vi "AlliGator Phasor Ratio Step.vi"(4 "Interactive?":bool, 6 "Time Stamp":dbl, 7 "Current Phasor Refnum":refnum<vi>, 8 "Error In":errorcluster, 10 "Phasor Ratio Parameters":T2, 11 "Registered Events Ctrl Refnums":T1) -> (0 "Error Out":errorcluster, 3 "Notebook String":string)   [LabVIEW 2021, in "AlliGator Phasor Ratio.lvlib"]
doc: "Computes phasor ratio and updates graphs."
uses:
  AlliGator Phasor Ratio.lvlib
  AlliGator Phasor Ratio Parameters.ctl
  Phasor/Phasor (g, s).ctl
  GUI/AlliGator Registered Events Ctrl Refnums.ctl
  Settings/AlliGator Settings List.ctl
  Graphs/XY Graph/XY Graph Plot Shift Parameters.ctl
  Graphs/XY Graph/XY Graph Plot Shift Method.ctl
  Phasor/Phasor Ratio Type.ctl
  Phasor/Phasor Standard Deviation Options.ctl
  Phasor/Phasor.lvlib
  Graphs/XY Graph/XY Graph Add-Ons.lvlib
  Settings/AlliGator Settings.lvlib
  Decay Analysis/Decay Preprocessing/AlliGator Decay Preprocessing.lvlib
  GUI/AlliGator GUI.lvlib
panel:
  in  "Data":variant
  # "see the AlliGator License on the block diagram (Ctrl+E or Window:Show Block Diagram)"
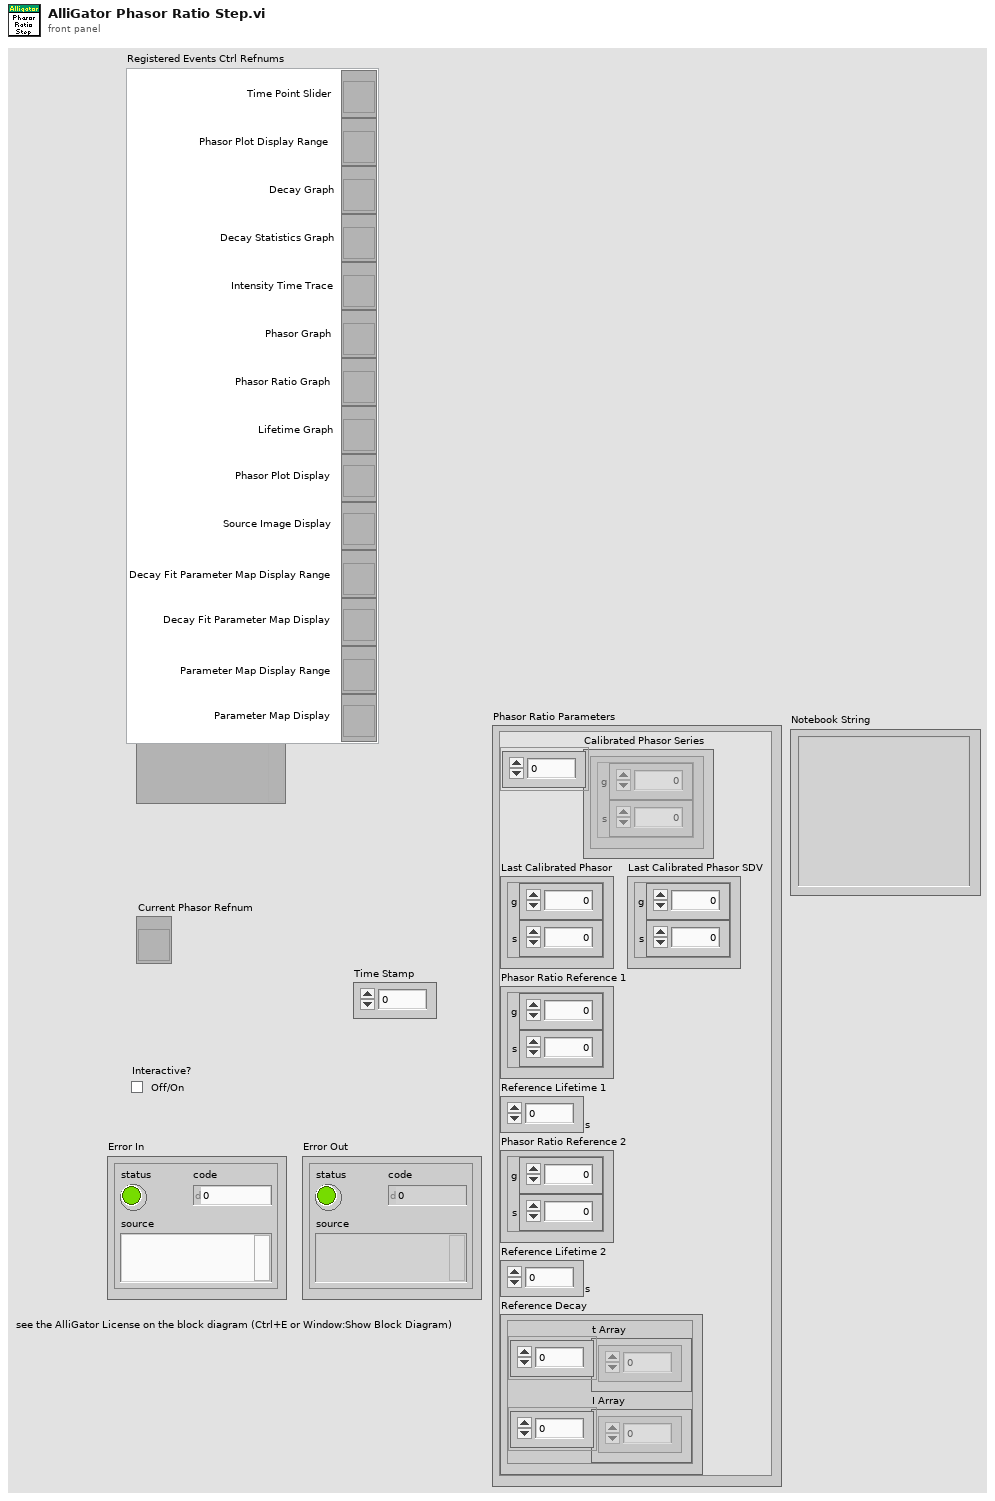
[diagram p1: front panel]
types:
  T1 = typedef "AlliGator GUI.lvlib/AlliGator Registered Events Ctrl Refnums.ctl" = cluster{"Time Point Slider":refnum<vi>, "Phasor Plot Display Range":refnum<vi>, "Decay Graph":refnum<vi>, "Decay Statistics Graph":refnum<vi>, "Intensity Time Trace":refnum<vi>, "Phasor Graph":refnum<vi>, "Phasor Ratio Graph":refnum<vi>, "Lifetime Graph":refnum<vi>, "Phasor Plot Display":refnum<vi>, "Source Image Display":refnum<vi>, "Decay Fit Parameter Map Display Range":refnum<vi>, "Decay Fit Parameter Map Display":refnum<vi>, "Parameter Map Display Range":refnum<vi>, "Parameter Map Display":refnum<vi>}
  T2 = typedef "AlliGator Phasor Ratio.lvlib/AlliGator Phasor Ratio Parameters.ctl" = cluster{"Calibrated Phasor Series":T3[], "Last Calibrated Phasor":T3, "Phasor Ratio Reference 1":T3, "Reference Lifetime 1":dbl[unit], "Phasor Ratio Reference 2":T3, "Reference Lifetime 2":dbl[unit], "Reference Decay":cluster{"t Array":dbl[], "I Array":dbl[]}, "Last Calibrated Phasor SDV":T3}
  T3 = typedef "Phasor.lvlib/Phasor (g, s).ctl" = cluster{"g":dbl, "s":dbl}
  T4 = typedef "XY Graph Add-Ons.lvlib/XY Graph Plot Shift Parameters.ctl" = cluster{"Type":T5, "Shift":dbl[unit], "Threshold":dbl, "Rotate":bool}
  T5 = typedef "XY Graph Add-Ons.lvlib/XY Graph Plot Shift Method.ctl" = enum16{"Default", "CFD", "Threshold", "Cross-Correlation"}
  T6 = typedef "AlliGator Settings.lvlib/AlliGator Settings List.ctl" = enum16{"GUI:Visible Settings Tab", "GUI:Last Run Version", "Source Image:Use Image Histogram for Contrast", "Source Image:Low Count Pixels Rejection Options", "Source Image:High Count Pixels Rejection Options", "Source Image:Use Image Brightness", "Source Image:Blend Overlay with Image Background", "Source Image:Use Fixed ROI Diameter", "Source Image:ROI Diameter", "Source Image:ROI Center Color", "Source Image:Peak Threshold", "Source Image:Intensity Threshold", "Source Image:Image Binning Options", "Source Image:Image Smoothing Options", "Source Image:Image Histogram Active", "Source Image:Invert Binary Mask", "Source Image:Hot Pixel Removal", "Source Image:Overlay Analyzed ROI Center", "Source Image:Auto-Adjust Contrast", "Source Image:Histogram Lower Percentile", "Source Image:Histogram Upper Percentile", "Source Image:Save Source Image", "Source Image:Scale Bar Options", "Source Image:Image Resolution (Pixel Size)", "Source Image:Flatfield Correction", "Source Image:Show Dead Left Columns Correction", "Source Image:Dead Left Columns Correction", "Source Image:Image Pre-Processing Operations Order", "Source Image:Overlay ROI Median", "Source Image:Median Overlay Color", "Data Information:Gate Width", "Data Information:Nanotime Gate Separation", "Data Information:Macrotime Gate Separation", "Data Information:Gate Step", "Data Information:# Gates", "Data Information:Gate Image Exposure", "Data Information:Gate Image Integration", "Data Information:Gates to Skip", "Data Information:Gates to Keep", "Data Information:Define Gates to", "Data Information:Channel Name", "Data Information:Available Channel Names", "Data Information:Channel Arithmetic", "Data Information:Background File Subtraction", "Data Information:Background File", "Data Information:Background Scaling Factor", "Data Information:Background Pile-up Correction", "Data Information:Background Pixel Well Capacity", "Data Information:Laser Period", "Data Information:SYNC Period", "Data Information:Pile-up Correction", "Data Information:Pixel Well Capacity", "Data Information:Dataset Scaling Factor", "Fluorescence Decay_Decay Pre-Processing:Reverse Gates", "Fluorescence Decay_Decay Pre-Processing:Verbose Decay Pre-Processing", "Fluorescence Decay_Decay Pre-Processing:Use Decay Pre-Processing", "Fluorescence Decay_Decay Pre-Processing:Background Subtraction", "Fluorescence Decay_Decay Pre-Processing:Background Definition Range", "Fluorescence Decay_Decay Pre-Processing:Baseline Subtraction Method", "Fluorescence Decay_Decay Pre-Processing:Decay Pre-Processing Operations Order", "Fluorescence Decay_Decay Pre-Processing:Smoothing Parameter", "Fluorescence Decay_Decay Pre-Processing:Shift Decay", "Fluorescence Decay_Decay Pre-Processing:Decay Shift Parameters", "Fluorescence Decay_Decay Pre-Processing:Fold Decay", "Fluorescence Decay_Decay Pre-Processing:# Folds", "Fluorescence Decay_Decay Pre-Processing:1-Normalize Decay", "Fluorescence Decay_Decay Pre-Processing:[0-1]-Normalize Decay", "Fluorescence Decay_Decay Pre-Processing:Smoothen Decay", "Fluorescence Decay_Decay Pre-Processing:Extrapolate Decay", "Fluorescence Decay_Decay Pre-Processing:Use Periodicity", "Fluorescence Decay_Decay Pre-Processing:Use Cursors", "Fluorescence Decay_Decay Pre-Processing:Tail Fraction", "Fluorescence Decay_Decay Pre-Processing:Head Fraction", "Fluorescence Decay_Decay Pre-Processing:Additional Points", "Fluorescence Decay_Decay Pre-Processing:Straighten Decay", "Fluorescence Decay_Decay Pre-Processing:Constant Background", "Fluorescence Decay_Decay Pre-Processing:Pixel-Normalize Decay", "Fluorescence Decay_Advanced Analysis:Extract IRF instead of Decay", "Fluorescence Decay_Advanced Analysis:IRF Extraction Options", "Fluorescence Decay_Advanced Analysis:IRF Optimization Options", "Fluorescence Decay_Advanced Analysis:Square Pulse Options", "Fluorescence Decay_Advanced Analysis:IRF Order", "Fluorescence Decay_Advanced Analysis:IRF Time Constants", "Fluorescence Decay_Advanced Analysis:Wavelet Analysis Options", "Fluorescence Decay_Advanced Analysis:Average Lifetime Options", "Fluorescence Decay_Fit Options:Fit Options", "Fluorescence Decay_Fit Options:Use Legacy Fitting Approach", "Fluorescence Decay_Fit Options:Use Data Information Laser Period", "Fluorescence Decay_Fit Parameters:Displayed Fit Parameters", "Fluorescence Decay_Fit Parameters:Fit Parameter Constraints", "Fluorescence Decay_Fit Parameters:Export Tabulated Results", "Fluorescence Decay_Fit Parameters:MLE Baseline Offset Type", "Fluorescence Decay_Fit Parameters:MLE Baseline Offset", "Fluorescence Decay_Fit Parameters:Guess Parameter Names", "Fluorescence Decay_Fit Parameters:Guess Parameter Values", "Fluorescence Decay_Fit Parameters:Guess Parameters Options", "Fluorescence Decay_Styles:Show Last Decay Only", "Fluorescence Decay_Styles:Decay Graph Color Array", "Fluorescence Decay:Decay Graph Active", "Fluorescence Decay Statistics:Min Peak Value", "Fluorescence Decay Statistics:Reject Low Decay Peak Pixels", "Fluorescence Decay Statistics:Reject High Decay Peak Pixels", "Fluorescence Decay Statistics:Max Peak Value", "Time Traces:Use File Timestamp", "Time Traces:Time Step", "Time Traces:Use Intensity Correction File", "Time Traces:Intensity Correction File", "Phasor Plot:Phasor Plot Smoothing Options", "Phasor Plot:Phasor Plot Size", "Phasor Plot:Phasor Plot Graphics Options", "Phasor Plot:Cumulative Phasor Plot", "Phasor Plot:Use Phasor Brightness", "Phasor Plot:Blend Overlay with Phasor Background", "Phasor Plot:Save Phasor Plot", "Phasor Plot:Show References", "Phasor Plot:Phasor Ratio Decay Range", "Phasor Plot:Exponential Fading", "Phasor Plot:Phasor Ratio Reference Colors", "Phasor Plot:Reference Radius", "Phasor Plot:Show Color Map Vertices", "Phasor Plot:Phasor Plot Active", "Phasor Plot:Phasor Ratio Color Map Type", "Phasor Plot:Phasor Ratio Color Map", "Phasor Plot:Phasor Ratio Display Range", "Phasor Plot:Selected Image ROI(s)", "Phasor Plot:All Image ROIs", "Phasor Plot:Selected Phasor Plot ROI(s)", "Phasor Plot:All Phasor Plot ROIs", "Phasor Plot:Phasor Ratio Color-Coded Quantity", "Phasor Plot:Store Phasor Harmonics", "Phasor Plot:Draw Reference Segment", "Phasor Plot:User-Defined Quantity", "Phasor Graph:Phasor Frequency", "Phasor Graph:Phasor Ratio Type", "Phasor Graph:Pixel-level Phasor Computation", "Phasor Graph:Save Phasor Graph", "Phasor Graph:Phasor Graph Active", "Phasor Graph:Phasor SDV Options", "Phasor Calibration:Use Backup Calibration if needed", "Phasor Graph:Define Shortest Lifetime as", "Phasor Calibration:Backup Calibration Type", "Phasor Calibration:Calibration Type", "Phasor Calibration:Calibration Lifetime", "Phasor Calibration:Calibration Map Algorithm", "Single-Exponential Phasor Locus (SEPL):Gate Parameters", "Single-Exponential Phasor Locus (SEPL):User-defined Gate", "Single-Exponential Phasor Locus (SEPL):User-defined IRF", "Single-Exponential Phasor Locus (SEPL):Phasor Parameters", "Single-Exponential Phasor Locus (SEPL):Decay & IRF Parameters", "Single-Exponential Phasor Locus (SEPL):Display Parameters", "Lifetime Analysis:Decay Analysis Parameters", "Lifetime Analysis:Lifetime Map Active", "Plugins:Python Settings", "Miscellaneous:Verbose Mode", "Miscellaneous:Beep after Script", "Miscellaneous:Saved Image File Format", "Miscellaneous:Exported Gate Image Settings", "Miscellaneous:Include Loading in Timing", "Miscellaneous:Verbose Settings Mode", "Miscellaneous:Histogram Options", "Miscellaneous:Beep on Error", "Miscellaneous:# Logical Processors Used", "Miscellaneous:ROI Description Max Characters", "Miscellaneous:Verbose Error Mode", "Miscellaneous:Transparent Mask Color"}
  T7 = typedef "Phasor.lvlib/Phasor Standard Deviation Options.ctl" = cluster{"Compute Estimated SDV":bool, "# Replicas":u32, "Use Estimated Average Phasor":bool}
  T8 = typedef "Phasor.lvlib/Phasor Ratio Type.ctl" = enum32{"Intensity-weighted", "Amplitude-weighted"}
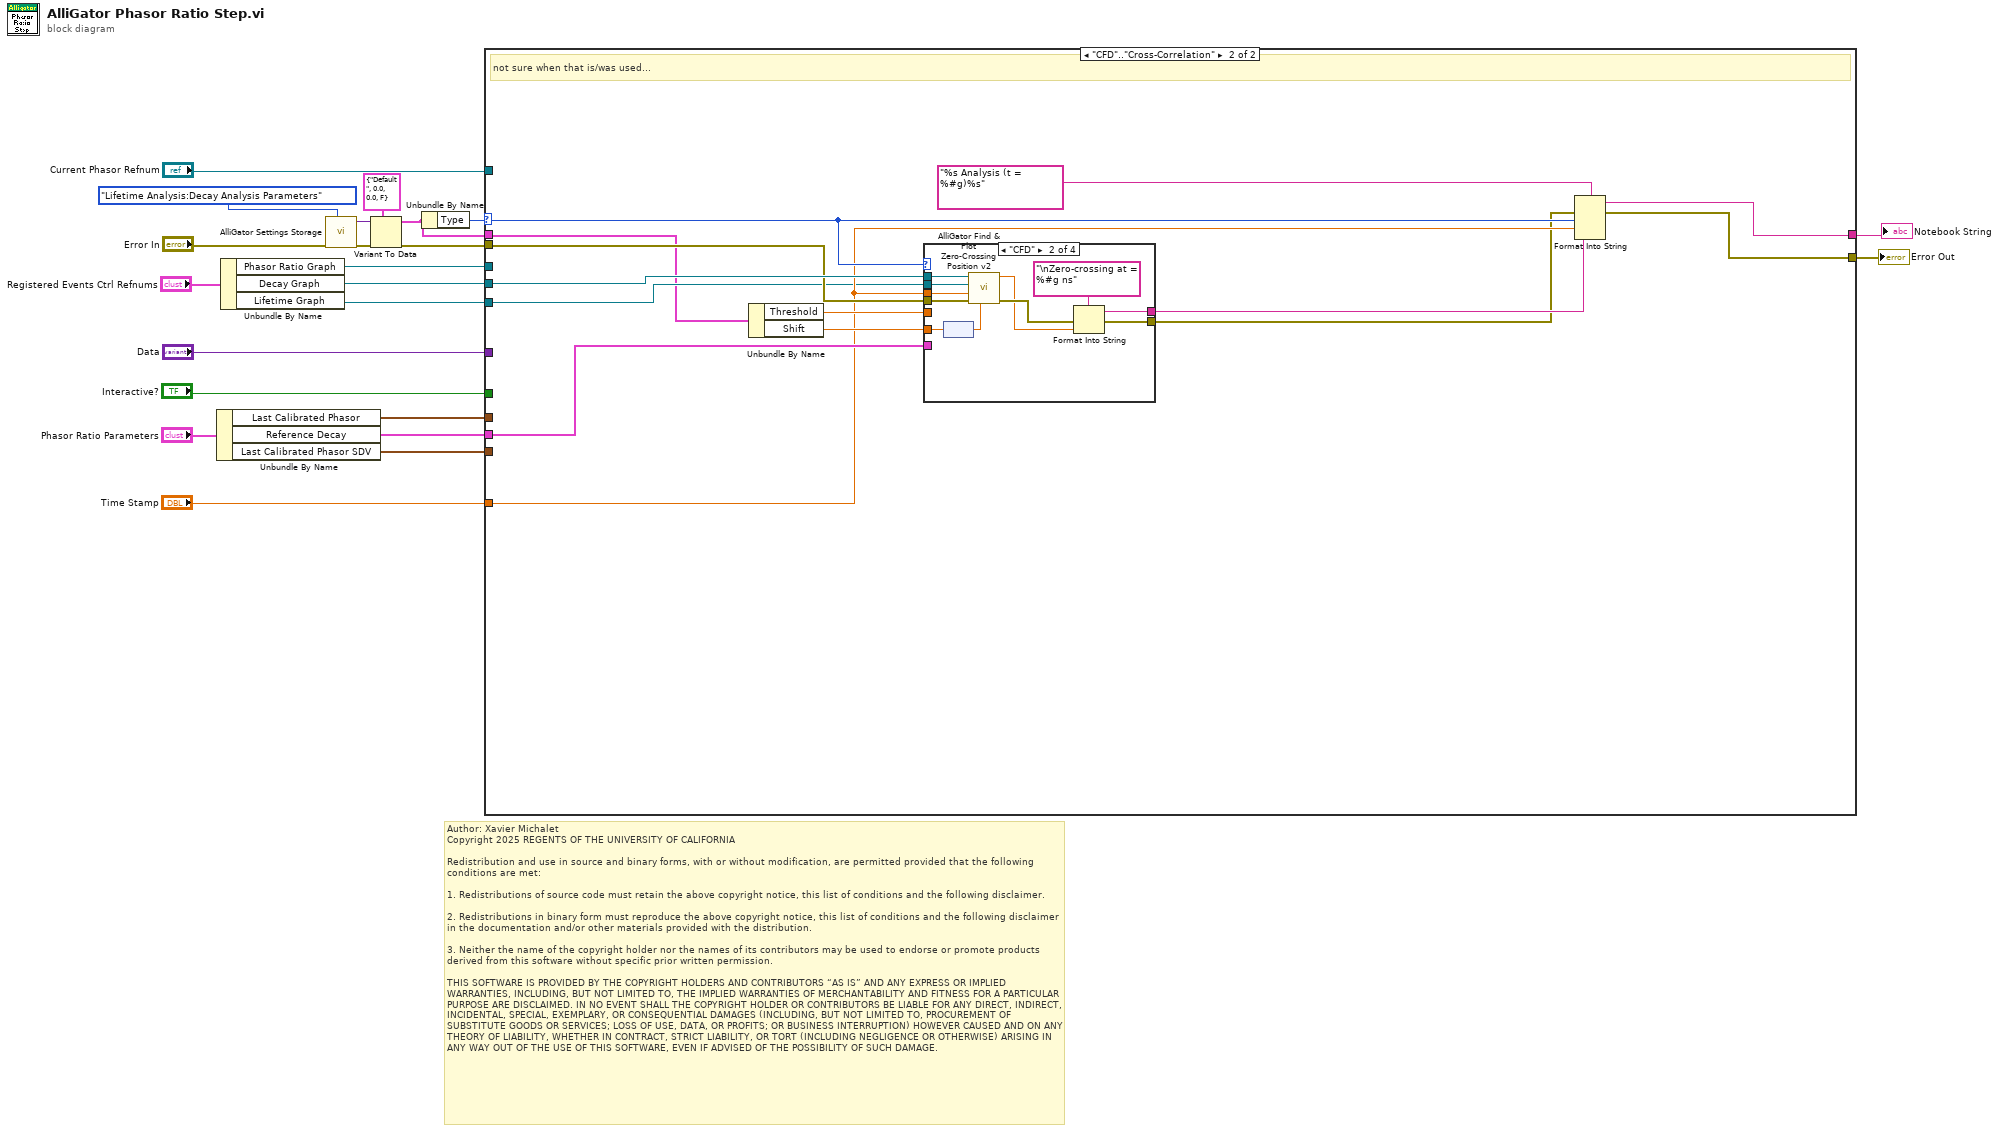
[diagram p0: block diagram]
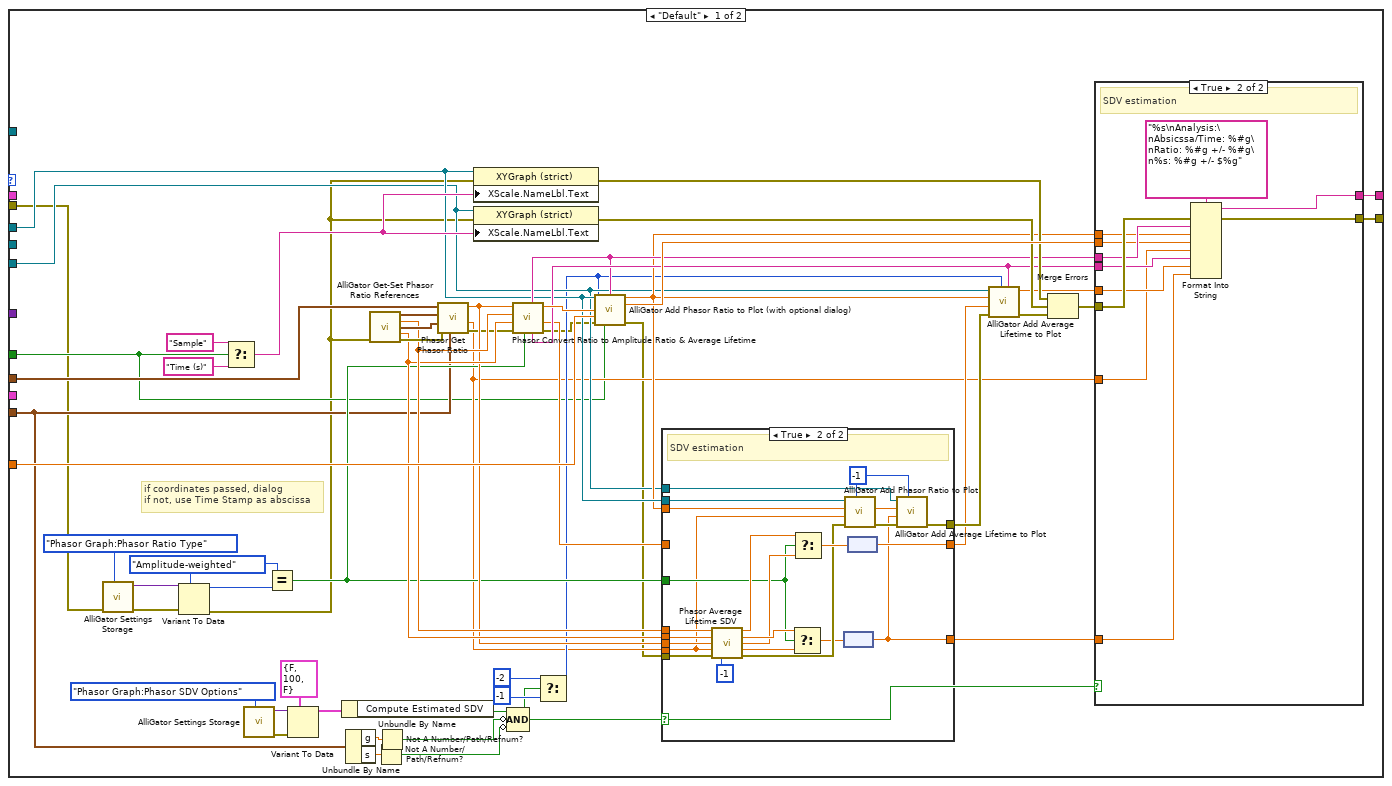
[diagram p2: hidden frame]
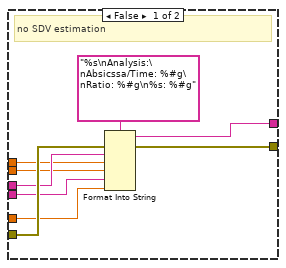
[diagram p3: hidden frame]
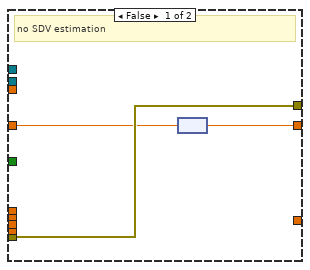
[diagram p4: hidden frame]
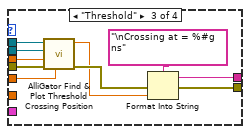
[diagram p6: hidden frame]
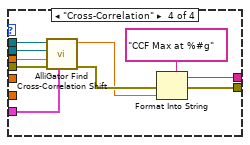
[diagram p7: hidden frame]
diagram:
  # "Author: Xavier Michalet\nCopyright 2025 REGENTS OF THE UNIVERSITY OF CALIFORNIA\n\nRedistribution and use in source and binary forms, with or without modification, are permitted provided that the following conditions are met:\n\n1. Redistributions of source code must retain the above copyright notice, this list of conditions and the following disclaimer.\n\n2. Redistributions in binary form must reproduce the above copyright notice, this list of conditions and the following disclaimer in the documentation and/or other materials provided with the distribution.\n\n3. Neither the name of the copyright holder nor the names of its contributors may be used to endorse or promote products derived from this software without specific prior written permission.\n\nTHIS SOFTWARE IS PROVIDED BY THE COPYRIGHT HOLDERS AND CONTRIBUTORS “AS IS” AND ANY EXPRESS OR IMPLIED WARRANTIES, INCLUDING, BUT NOT LIMITED TO, THE IMPLIED WARRANTIES OF MERCHANTABILITY AND FITNESS FOR A PARTICULAR PURPOSE ARE DISCLAIMED. IN NO EVENT SHALL THE COPYRIGHT HOLDER OR CONTRIBUTORS BE LIABLE FOR ANY DIRECT, INDIRECT, INCIDENTAL, SPECIAL, EXEMPLARY, OR CONSEQUENTIAL DAMAGES (INCLUDING, BUT NOT LIMITED TO, PROCUREMENT OF SUBSTITUTE GOODS OR SERVICES; LOSS OF USE, DATA, OR PROFITS; OR BUSINESS INTERRUPTION) HOWEVER CAUSED AND ON ANY THEORY OF LIABILITY, WHETHER IN CONTRACT, STRICT LIABILITY, OR TORT (INCLUDING NEGLIGENCE OR OTHERWISE) ARISING IN ANY WAY OUT OF THE USE OF THIS SOFTWARE, EVEN IF ADVISED OF THE POSSIBILITY OF SUCH DAMAGE."
  n1 = Unbundle By Name("Phasor Ratio Parameters") -> ("Last Calibrated Phasor"=w16:T3, "Reference Decay"=w15:cluster{"t Array":dbl[], "I Array":dbl[]}, "Last Calibrated Phasor SDV"=w2:T3)
  n2 = Unbundle By Name("Registered Events Ctrl Refnums") -> ("Phasor Ratio Graph"=w17:refnum<vi>, "Decay Graph"=w19:refnum<vi>, "Lifetime Graph"=w18:refnum<vi>)
  n3 = call "AlliGator Settings Storage.vi"("AlliGator Settings List"=AlliGator_Settings_List."Lifetime Analysis:Decay Analysis Parameters", "Error In"="Error In") -> ("Error Out"=w5:errorcluster, "Variant Data out"=w11:variant)  [unwired: 8 in]
  n4 = Variant To Data(error in=w5, type=T4 {"Type"=enum."Default", "Shift"=0.0, "Threshold"=0.0, "Rotate"=FALSE} ("IRF Analysis Method"), Variant=w11) -> (data=w7:T4, error out=w4:errorcluster)
  n5 = Unbundle By Name(w7) -> ("Type"=w10:T5)
  n6 = case shown="\"CFD\"..\"Cross-Correlation\"" w10 {
    selector: w10 -> [_ w133]
    tunnel: "Data" -> [_ _]
    tunnel: w16 -> [w52 _]
    tunnel: w15 -> [_ w138]
    tunnel: "Time Stamp" -> [w76 w131]
    tunnel: w17 -> [w42 _]
    tunnel: w19 -> [_ w135]
    tunnel: "Current Phasor Refnum" -> [_ _]
    tunnel: w18 -> [w40 w128]
    tunnel: [w71 w125] -> w13
    tunnel: w4 -> [w25 w134]
    tunnel: [w78 w130] -> w8
    tunnel: w7 -> [_ w127]
    tunnel: w2 -> [w45 _]
    tunnel: "Interactive?" -> [w29 _]
    frame "Default" {
      w64 = Phasor_Ratio_Type."Amplitude-weighted" ("Phasor Ratio Type")
      # "if coordinates passed, dialog\nif not, use Time Stamp as abscissa"
      n7 = call "AlliGator Settings Storage.vi"("AlliGator Settings List"=AlliGator_Settings_List."Phasor Graph:Phasor Ratio Type", "Error In"=w25) -> ("Error Out"=w62:errorcluster, "Variant Data out"=w63:variant)  [unwired: 8 in]
      n8 = Variant To Data(error in=w62, type=w64, Variant=w63) -> (data=w65:T8, error out=w26:errorcluster)
      n9 = Select(t="Sample" ("X Scale.Name Label.Text"), s=w29, f="Time (s)") -> (s? t:f=w79:string)
      n10 = call "AlliGator Settings Storage.vi"("AlliGator Settings List"=AlliGator_Settings_List."Phasor Graph:Phasor SDV Options") -> ("Error Out"=w58:errorcluster, "Variant Data out"=w60:variant)  [unwired: 9 in]
      n11 = Equal?(x=w64, y=w65) -> (x = y?=w46:bool)
      n12 = Variant To Data(error in=w58, type=T7 {"Compute Estimated SDV"=FALSE, "# Replicas"=100, "Use Estimated Average Phasor"=FALSE} ("Phasor SDV Options"), Variant=w60) -> (data=w61:T7)  [unwired: 1 out]
      n13 = Unbundle By Name(w61) -> ("Compute Estimated SDV"=w56:bool)
      n14 = Unbundle By Name(w45) -> ("g"=w30:dbl, "s"=w57:dbl)
      n15 = call "AlliGator Get-Set Phasor Ratio References.vi"("error in (no error)"=w26) -> ("Reference Phasor 1"=w74:T3, "Reference Lifetime 1"=w51:dbl[unit], "Reference Phasor 2"=w73:T3, "Reference Lifetime 2"=w50:dbl[unit], "error out"=w72:errorcluster)  [unwired: 7 in, 3 out]
      n16 = Not A Number/Path/Refnum?(number/path/refnum=w57) -> (NaN/Path/Refnum?=w54:bool)
      n17 = Not A Number/Path/Refnum?(number/path/refnum=w30) -> (NaN/Path/Refnum?=w55:bool)
      n18 = call "Phasor Get Phasor Ratio.vi"("Phasor SDV"=w45, "Error In"=w72, "Reference Phasor 2"=w73, "Reference Phasor 1"=w74, "Phasor"=w52) -> ("Error Out"=w48:errorcluster, "Phasor Ratio SDV"=w32:dbl, "Phasor Ratio (f1)"=w49:dbl)  [unwired: 4 in]
      n19 = property class="XYGraph (strict)"(reference=w42, error in=w26, "XScale.NameLbl.Text"=w79) -> (error out=w69:errorcluster)  [unwired: 1 out]
      n20 = property class="XYGraph (strict)"(reference=w40, error in=w26, "XScale.NameLbl.Text"=w79) -> (error out=w70:errorcluster)  [unwired: 1 out]
      n21 = Compound Arithmetic op=AND(w56, invert w55, invert w54) -> (w33:bool)
      n22 = call "Phasor Convert Ratio to Amplitude Ratio & Average Lifetime.vi"("Compute Amplitude Ratio"=w46, "error in (no error)"=w48, "Reference Lifetime 2"=w50, "Reference Lifetime 1"=w51, "Phasor Ratio (f1)"=w49) -> ("error out"=w24:errorcluster, "Average Lifetime"=w47:dbl[unit], "Phasor/Amplitude Ratio"=w77:dbl, "Average Lifetime Caption"=w68:string, "Phasor Ratio Plot Name Suffix"=w67:string)  [unwired: 2 in]
      n23 = Select(t=-2 ("Plot ID (-1)"), s=w33, f=-1 ("Plot ID (-1)")) -> (s? t:f=w34:i32)
      n24 = call "AlliGator Add Phasor Ratio to Plot (with optional dialog).vi"("XYGraph in"=w42, "Plot ID (-1)"=w34, "Phasor Ratio"=w77, "Time Point"=w76, "error in (no error)"=w24, "Interactive?"=w29, "New Plot Name"=w67) -> ("Sample Abscissa"=w41:dbl, "Phasor Ratio"=w75:dbl, "error out"=w23:errorcluster)  [unwired: 3 in, 3 out]
      n25 = case shown="True" w33 {
        tunnel: w23 -> [w102 w119]
        tunnel: w51 -> [_ w124]
        tunnel: w50 -> [_ w123]
        tunnel: [w102 w110] -> w39
        tunnel: w32 -> [_ w112]
        tunnel: w49 -> [_ w122]
        tunnel: w46 -> [_ w115]
        tunnel: w47 -> [w100 _]
        tunnel: [w101 w105] -> w35
        tunnel: w42 -> [_ w114]
        tunnel: w41 -> [_ w108]
        tunnel: w40 -> [_ w106]
        tunnel: [_ w104] -> w31
        frame False {
          # "no SDV estimation"
          n26 = node(w100) -> (w101:dbl)
        }
        frame True {
          w109 = -1 ("Plot ID (-1)")
          # "SDV estimation"
          n27 = call "Phasor Average Lifetime SDV.vi"("tau 1"=w124, "tau 2"=w123, "r"=w122, "SDV r"=w112, "Error In"=w119, "seed"=-1) -> ("<tau>_a"=w118:dbl[unit], "SDV <tau>_a"=w121:dbl[unit], "<tau>_i"=w117:dbl[unit], "SDV <tau>_i"=w120:dbl[unit], "Error Out"=w113:errorcluster)  [unwired: 4 in, 1 out]
          n28 = Select(t=w121, s=w115, f=w120) -> (s? t:f=w107:dbl[unit])
          n29 = Select(t=w118, s=w115, f=w117) -> (s? t:f=w116:dbl[unit])
          n30 = node(w107) -> (w104:dbl)
          n31 = call "AlliGator Add Phasor Ratio to Plot.vi"("Plot ID (-1)"=w109, "error in (no error)"=w113, "Phasor Ratio"=w112, "Abscissa"=w108, "Phasor Ratio Graph refnum"=w114) -> ("error out"=w111:errorcluster)  [unwired: 3 in, 3 out]
          n32 = node(w116) -> (w105:dbl)
          n33 = call "AlliGator Add Average Lifetime to Plot.vi"("Plot ID (-1)"=w109, "error in (no error)"=w111, "Average Lifetime"=w104, "Abscissa"=w108, "Lifetime Graph refnum"=w106) -> ("error out"=w110:errorcluster)  [unwired: 3 in, 3 out]
        }
      }
      n34 = call "AlliGator Add Average Lifetime to Plot.vi"("New Plot Name"=w68, "Plot ID (-1)"=w34, "error in (no error)"=w39, "Average Lifetime"=w35, "Abscissa"=w41, "Lifetime Graph refnum"=w40) -> ("error out"=w38:errorcluster, "Average Lifetime (dup)"=w36:dbl)  [unwired: 2 in, 2 out]
      n35 = Merge Errors(w69, w70, w38) -> (w37:errorcluster)
      n36 = case shown="True" w33 {
        tunnel: w37 -> [w88 w99]
        tunnel: [w87 w98] -> w71
        tunnel: [w86 w97] -> w78
        tunnel: w67 -> [w84 w95]
        tunnel: w41 -> [w83 w94]
        tunnel: w75 -> [w82 w93]
        tunnel: w68 -> [w81 w92]
        tunnel: w36 -> [w80 w91]
        tunnel: w32 -> [_ w90]
        tunnel: w31 -> [_ w89]
        frame False {
          # "no SDV estimation"
          n37 = Format Into String(format string="%s\nAnalysis:\nAbsicssa/Time: %#g\nRatio: %#g\n%s: %#g", error in=w88, w84, w83, w82, w81, w80) -> (resulting string=w86:string, error out=w87:errorcluster)  [unwired: 1 in]
        }
        frame True {
          # "SDV estimation"
          n38 = Format Into String(format string="%s\nAnalysis:\nAbsicssa/Time: %#g\nRatio: %#g +/- %#g\n%s: %#g +/- $%g", error in=w99, w95, w94, w93, w90, w92, w91, w89) -> (resulting string=w97:string, error out=w98:errorcluster)  [unwired: 1 in]
        }
      }
    }
    frame "CFD".."Cross-Correlation" {
      # "not sure when that is/was used..."
      n39 = Unbundle By Name(w127) -> ("Threshold"=w137:dbl, "Shift"=w136:dbl[unit])
      n40 = case shown="\"CFD\"" w133 {
        tunnel: w128 -> [_ w150 w160 w170]
        tunnel: w135 -> [_ w149 w159 w169]
        tunnel: w138 -> [_ _ _ w168]
        tunnel: w131 -> [_ w148 w158 w167]
        tunnel: w137 -> [_ _ w155 _]
        tunnel: w136 -> [_ w147 _ _]
        tunnel: w134 -> [w139 w146 w157 w166]
        tunnel: [w139 w141 w152 w162] -> w126
        tunnel: [_ w143 w154 w164] -> w129
        frame "Default", Default {
          # "Handled in other main case"
        }
        frame "CFD" {
          n41 = node(w147) -> (w144:dbl)
          n42 = call "AlliGator Find & Plot Zero-Crossing Position v2.vi"("Shift"=w144, "Error In"=w146, "Time Stamp"=w148, "Lifetime Graph"=w150, "Decay Graph"=w149) -> ("Error Out"=w142:errorcluster, "Zero Position"=w140:dbl)  [unwired: 5 in]
          n43 = Format Into String(format string="\nZero-crossing at = %#g ns", error in=w142, w140) -> (resulting string=w143:string, error out=w141:errorcluster)  [unwired: 1 in]
        }
        frame "Threshold" {
          n44 = call "AlliGator Find & Plot Threshold Crossing Position.vi"("Threshold"=w155, "Error In"=w157, "Time Stamp"=w158, "Lifetime Graph"=w160, "Decay Graph"=w159) -> ("Error Out"=w153:errorcluster, "Crossing Position"=w151:dbl)  [unwired: 5 in]
          n45 = Format Into String(format string="\nCrossing at = %#g ns", error in=w153, w151) -> (resulting string=w154:string, error out=w152:errorcluster)  [unwired: 1 in]
        }
        frame "Cross-Correlation" {
          n46 = call "AlliGator Find Cross-Correlation Shift.vi"("Reference Decay"=w168, "Error In"=w166, "Time Stamp"=w167, "Lifetime Graph"=w170, "Decay Graph"=w169) -> ("Error Out"=w163:errorcluster, "Zero Position"=w161:dbl)  [unwired: 5 in]
          n47 = Format Into String(format string="CCF Max at %#g", error in=w163, w161) -> (resulting string=w164:string, error out=w162:errorcluster)  [unwired: 1 in]
        }
      }
      n48 = Format Into String(format string="%s Analysis (t = %#g)%s", error in=w126, w133, w131, w129) -> (resulting string=w130:string, error out=w125:errorcluster)  [unwired: 1 in]
    }
  }
  "Error Out" <- w13
  "Notebook String" <- w8
